vi "AddClusterCtls.vi"(8 "error IO In":errorcluster, 11 "CtlLookup In":T1) -> (0 "error IO":errorcluster, 3 "CtlLookup Out":T1)   [LabVIEW 2024, in "CtlReferences.lvlib" / "CtlReferences.lvclass"]
doc: "Add all cluster (and subcluster) element control refs\nto the DVR ctl storage. -- Cluster names are specified by ClusterName.ControlName"
uses:
  CtlReferences.lvclass
  TypeDefs/CtlLookup.ctl
  CtlReferences.lvclass/CtlReferences.ctl
  AddControl.vi
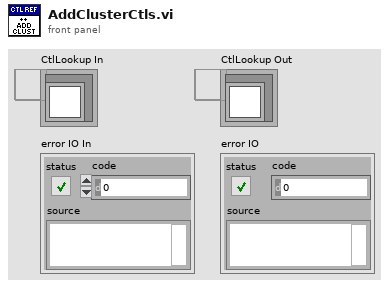
[diagram p1: front panel]
types:
  T1 = typedef "CtlReferences.lvlib/CtlReferences.lvclass/CtlLookup.ctl" = refnum<data-value>
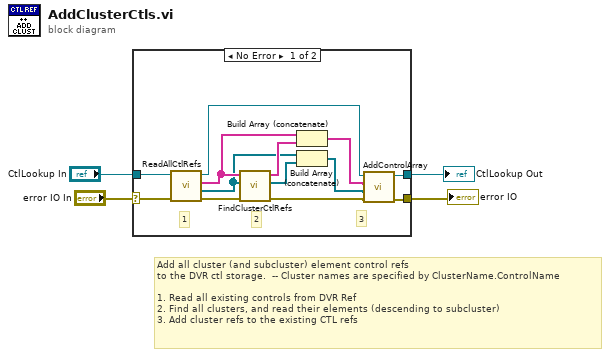
[diagram p0: block diagram]
diagram:
  # "Add all cluster (and subcluster) element control refs\nto the DVR ctl storage.  -- Cluster names are specified by ClusterName.ControlName\n\n1. Read all existing controls from DVR Ref\n2. Find all clusters, and read their elements (descending to subcluster)\n3. Add cluster refs to the existing CTL refs"
  n1 = case shown="No Error" "error IO In" {
    selector: "error IO In" -> [w15 w19]
    tunnel: "CtlLookup In" -> [w17 w18]
    tunnel: [w9 w18] -> w2
    tunnel: [w10 w19] -> w1
    frame No Error {
      # "3"
      # "2"
      # "1"
      n2 = call "ReadAllCtlRefs.vi"("error in (no error)"=w15, "CtlLookup In"=w17) -> ("error out"=w16:errorcluster, "CtlRef Array"=w11:refnum<vi>[], "CtlName Array"=w12:string[], "CtlLookup Out"=w8:T1)  [unwired: 6 in]
      n3 = call "FindClusterCtlRefs.vi"("error in (no error)"=w16, "CLT Ref Array"=w11, "CTL Name Array"=w12) -> ("error out"=w5:errorcluster, "Cluster CTL Array"=w14:refnum<vi>[], "Cluster CTL Name Array"=w13:string[])  [unwired: 6 in]
      n4 = Build Array (concatenate)(w12, w13) -> (w7:string[])
      n5 = Build Array (concatenate)(w11, w14) -> (w6:refnum<vi>[])
      n6 = call "AddControlArray.vi"("error in (no error)"=w5, "CtlRef Array"=w6, "CtlLabel Array"=w7, "CtlLookup In"=w8) -> ("error out"=w10:errorcluster, "CtlLookup Out"=w9:T1)  [unwired: 6 in]
    }
    frame Error {
    }
  }
  "error IO" <- w1
  "CtlLookup Out" <- w2
